vi "ArmSequencer.vi"(0 "Reset":bool, 3 "Array of Arm Joint Goals":cluster{dbl, dbl, dbl}[](array[cluster]), 5 "Treat Wrist as Four-Bar":bool) -> (8 "Current Sequence Step":i32, 9 "Arm Has Arrived":bool, 14 "Goal Shoulder Angle (deg)":dbl, 15 "Goal Elbow Angle (deg)":dbl, 16 "Goal Wrist Angle (deg)":dbl, 17 "Shoulder Control Mode":T1(ring), 18 "Elbow Control Mode":T1(ring), 19 "Wrist Control Mode":T1(ring))   [LabVIEW 2020]
doc: "Sequences the arm joint angles using an array of clusters specifiying waypoints. The last waypoint uses the positioning control mode while the intermediate waypoints are reached using the traveling control mode."
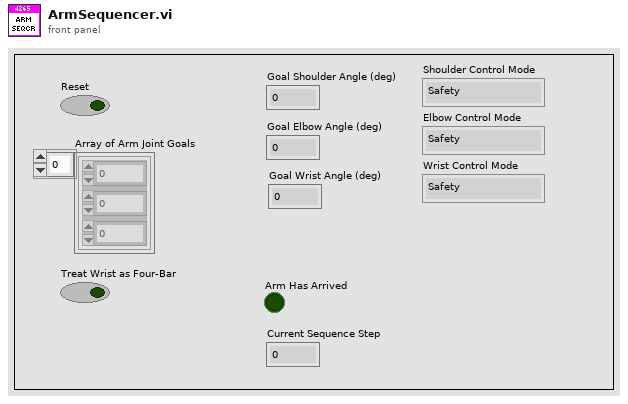
[diagram p1: front panel]
types:
  T1 = enum16{"Safety", "Travelling", "Positioning", "Holding"}
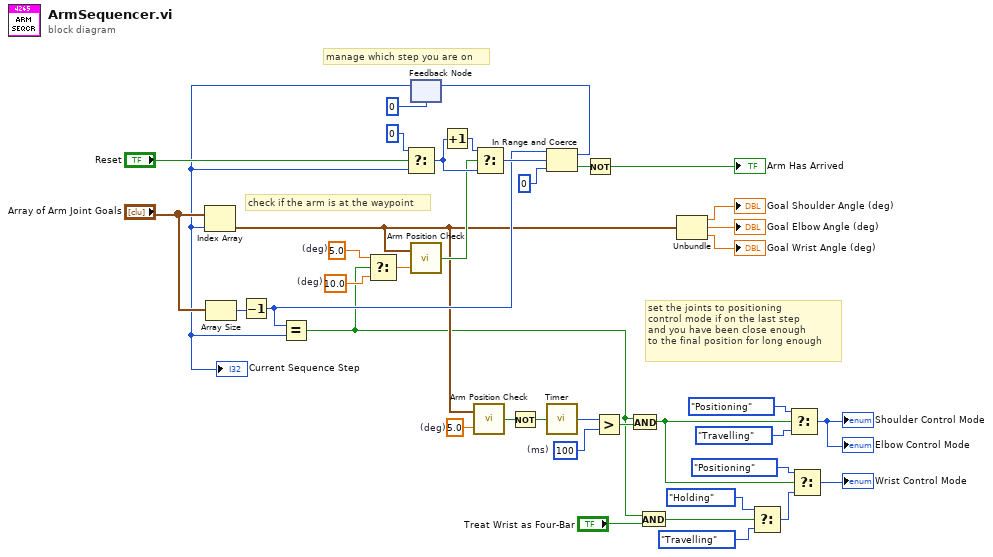
[diagram p0: block diagram]
diagram:
  w13 = u32 100  # (ms)
  w17 = 5.0  # (deg)
  w19 = 10.0  # (deg)
  w20 = 5.0  # (deg)
  # "check if the arm is at the waypoint"
  # "set the joints to positioning\ncontrol mode if on the last step\nand you have been close enough\nto the final position for long enough"
  # "manage which step you are on"
  n1 = Array Size(array="Array of Arm Joint Goals") -> (size(s)=w39:i32)
  n2 = Decrement(x=w39) -> (x-1=w24:i32)
  n3 = feedback #1(0) -> (w23:i32)
  "Current Sequence Step" <- w23
  n4 = Index Array(array="Array of Arm Joint Goals", index=w23) -> (element=w12:cluster{dbl, dbl, dbl})
  n5 = Equal?(x=w24, y=w23) -> (x = y?=w3:bool)
  n6 = Select(t=w20, s=w3, f=w19) -> (s? t:f=w18:dbl)
  n7 = Select(t=0, s="Reset", f=w23) -> (s? t:f=w40:i32)
  n8 = call "Arm Position Check.vi"("Threshold (deg)"=w18, "Goal Angles (deg)"=w12) -> ("Is Within Threshold"=w38:bool)
  n9 = Increment(x=w40) -> (x+1=w37:i32)
  n10 = call "Arm Position Check.vi"("Threshold (deg)"=w17, "Goal Angles (deg)"=w12) -> ("Is Within Threshold"=w16:bool)
  n11 = Select(t=w37, s=w38, f=w40) -> (s? t:f=w29:i32)
  n12 = Not(x=w16) -> (.not. x?=w15:bool)
  n13 = In Range and Coerce(upper limit=w24, x=w29, lower limit=0) -> (coerced(x)=w27:i32, In Range?=w26:bool)
  n14 = feedback-in #1(w27) -> ()
  n15 = call "Timer.vi"("Reset Timer"=w15) -> ("Time (ms)"=w14:u32)
  n16 = Not(x=w26) -> (.not. x?=→"Arm Has Arrived":bool)
  n17 = Greater?(x=w14, y=w13) -> (0:w11:bool)
  n18 = And(x=w3, y=w11) -> (x .and. y?=w8:bool)
  n19 = And(x=w3, y="Treat Wrist as Four-Bar") -> (x .and. y?=w1:bool)
  n20 = Unbundle(w12) -> (→"Goal Shoulder Angle (deg)":dbl, →"Goal Elbow Angle (deg)":dbl, →"Goal Wrist Angle (deg)":dbl)
  n21 = Select(t=T1."Holding", s=w1, f=T1."Travelling" ("OUT_Shoulder_Mode")) -> (s? t:f=w5:T1)
  n22 = Select(t=T1."Positioning" ("OUT_Shoulder_Mode"), s=w8, f=T1."Travelling" ("OUT_Shoulder_Mode")) -> (s? t:f=→"Shoulder Control Mode" →"Elbow Control Mode":T1)
  n23 = Select(t=T1."Positioning" ("OUT_Shoulder_Mode"), s=w8, f=w5) -> (s? t:f=→"Wrist Control Mode":T1)
